vi "testExtractTopicContents.vi"(8 "error in (no error)":errorcluster) -> (0 "error out":errorcluster)   [LabVIEW 2018]
uses:
  SALTypeGenerator/Module/Module.lvclass
  SALTypeGenerator/Module/Module.lvclass/Module.ctl
  <vilib>/addons/_JKI Toolkits/Caraya/classes/Assert/Assert Equal Value_Variant.vi
  <vilib>/addons/_JKI Toolkits/Caraya/classes/Test/Test.lvclass
  <vilib>/addons/_JKI Toolkits/Caraya/classes/Assert/Assert.lvclass
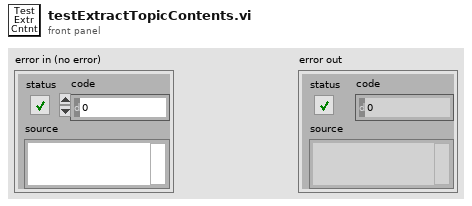
[diagram p1: front panel]
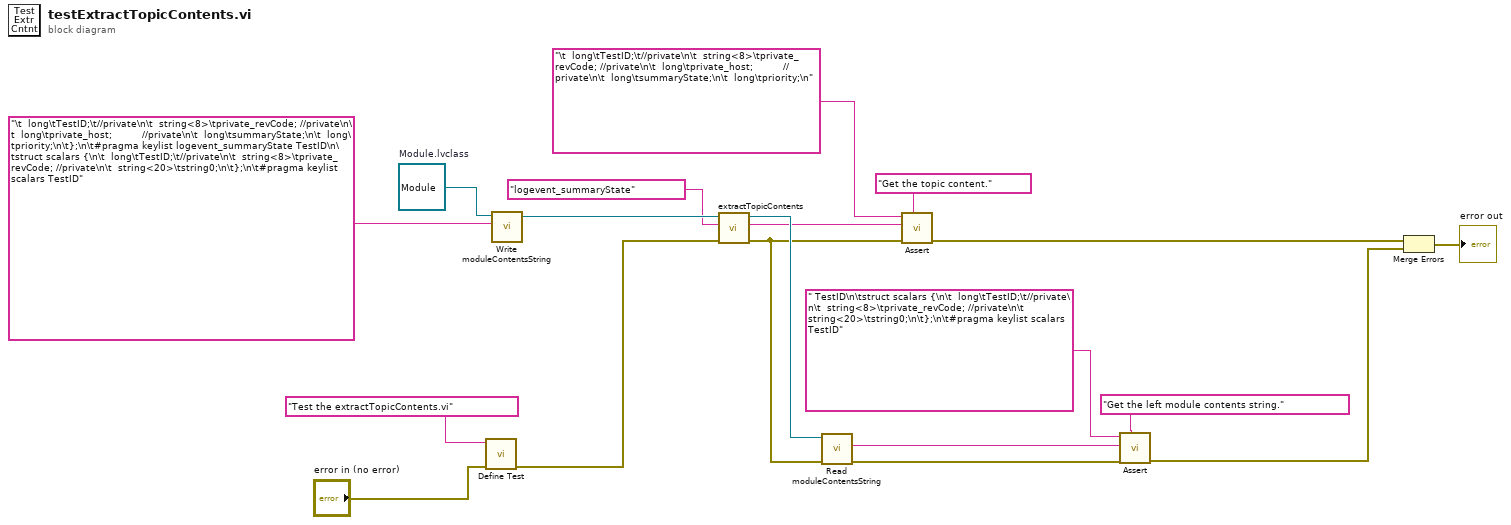
[diagram p0: block diagram]
diagram:
  w17 = refnum<class "Module.lvclass"> refnum  # Module.lvclass
  n1 = call <vilib>:"Define Test.vi"("error in (no error)"="error in (no error)", "Label (VI Title)"="Test the extractTopicContents.vi") -> ("error out"=w13:errorcluster)  [unwired: 9 in]
  n2 = call "Write moduleContentsString.vi"("moduleContentsString"="\t  long\tTestID;\t//private\n\t  string<8>\tprivate_revCode; //private\n\t  long\tprivate_host;          //private\n\t  long\tsummaryState;\n\t  long\tpriority;\n\t};\n\t#pragma keylist logevent_summaryState TestID\n\tstruct scalars {\n\t  long\tTestID;\t//private\n\t  string<8>\tprivate_revCode; //private\n\t  string<20>\tstring0;\n\t};\n\t#pragma keylist scalars TestID", "Module in"=w17) -> ("Module out"=w16:refnum<class "Module.lvclass">)  [unwired: 9 in]
  n3 = call "extractTopicContents.vi"("error in (no error)"=w13, "topicName"="logevent_summaryState", "Module in"=w16) -> ("error out"=w12:errorcluster, "topicContentsString"=w11:string, "Module out"=w14:refnum<class "Module.lvclass">)  [unwired: 6 in]
  n4 = call "Read moduleContentsString.vi"("error in (no error)"=w12, "Module in"=w14) -> ("error out"=w9:errorcluster, "moduleContentsString"=w8:string)  [unwired: 7 in, 1 out]
  n5 = call-poly <vilib>:"Assert.vi"("Label"="Get the topic content.", "error in (no error)"=w12, "Y"=w11, "X"="\t  long\tTestID;\t//private\n\t  string<8>\tprivate_revCode; //private\n\t  long\tprivate_host;          //private\n\t  long\tsummaryState;\n\t  long\tpriority;\n") -> ("error out"=w6:errorcluster)  [unwired: 7 in]
  n6 = call-poly <vilib>:"Assert.vi"("Label"="Get the left module contents string.", "error in (no error)"=w9, "Y"=w8, "X"=" TestID\n\tstruct scalars {\n\t  long\tTestID;\t//private\n\t  string<8>\tprivate_revCode; //private\n\t  string<20>\tstring0;\n\t};\n\t#pragma keylist scalars TestID") -> ("error out"=w5:errorcluster)  [unwired: 7 in]
  n7 = Merge Errors(w6, w5) -> (→"error out":errorcluster)
